vi "LSCI332 WaitSetpoint.vi"(0 "VISA Rsrc":refnum<visa-resource-name>="GPIB0::12::INSTR", 1 "ForceStop":refnum<vi>, 2 "Temp K":refnum<vi>, 3 "Heat":refnum<vi>, 5 "Wait Stab":bool=TRUE, 7 "SetPoint":dbl, 9 "Entré Activées":bool[](array[boolean])=[TRUE, FALSE], 11 "error in (no error)":errorcluster, 12 "Timeout":u32 caption="Timeout(s)", 13 "RangeK":dbl=0.01 min=0.01 max=100.0 step=0.01, 14 "InRangeTime":i32 caption="Req In Range Time(s)") -> (6 "TempOut (K)":dbl caption="Temp (K)", 8 "TempOut (S)":dbl, 15 "error out":errorcluster)   [LabVIEW 2019]
doc: "Ce VI écrit les paramètres limites de contrôle dans le contrôleur."
uses:
  <vilib>/Utility/error.llb/Error Cluster From Error Code.vi
  <userlib>/GenProg/ReadValByRefBool.vi
  <vilib>/ErrorRing/Error Ring.xnode
panel:
  in  "Open FP":bool
  in  "Force Stop":bool
  out "Elapsed Time(s)":u32 caption="Elapsed Time (s)" format="%<%H:%M>t"
  out "heating":bool
  out "Puissance(%)":dbl
  out "Échelle":u16
  out "Graphe XY":cluster{dbl[], dbl[]}[](graph)
  out "InRangeTimeOut":i32 caption="In Range Time (s)"
  out "In Range":bool
  in  "Boucle(1)":u32(ring) caption="Boucle" items=["Boucle 1", "Boucle 2"]
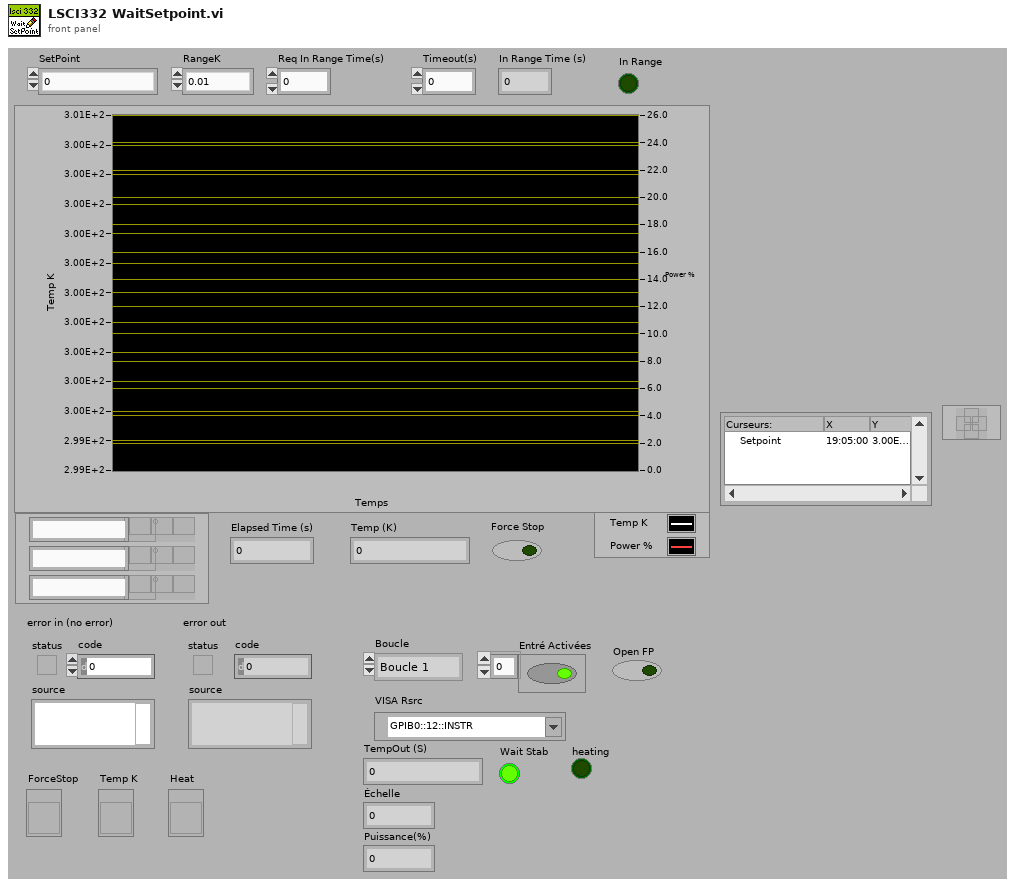
[diagram p1: front panel]
types:
  T1 = enum32{"Invalid", "Standard", "Closed", "Hidden", "Minimized", "Maximized"}
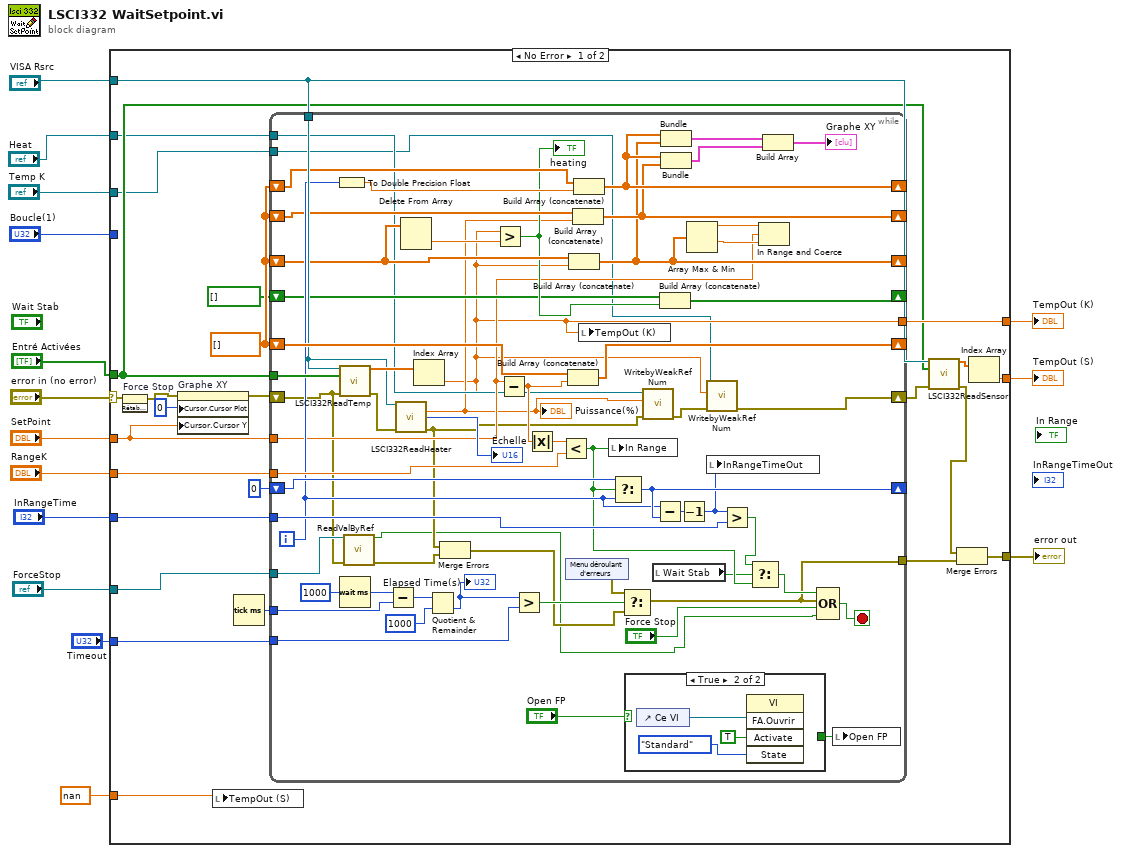
[diagram p0: block diagram]
diagram:
  n1 = case shown="No Error" "error in (no error)" {
    selector: "error in (no error)" -> [w22 w113]
    tunnel: "VISA Rsrc" -> [w34 _]
    tunnel: "Boucle(1)" -> [_ _]
    tunnel: [w30 w113] -> w13
    tunnel: "SetPoint" -> [w24 _]
    tunnel: "Entré Activées" -> [w31 _]
    tunnel: "Timeout" -> [w39 _]
    tunnel: "RangeK" -> [w38 _]
    tunnel: "InRangeTime" -> [w36 _]
    tunnel: [w35 _] -> w6
    tunnel: [w32 _] -> w5
    tunnel: nan ("TempOut (S)") -> [w28 _]
    tunnel: "ForceStop" -> [w16 _]
    tunnel: "Heat" -> [w18 _]
    tunnel: "Temp K" -> [w17 _]
    frame No Error {
      w27 = dbl[] []
      n2 = invoke on="Force Stop" class="Bool (strict)" method="RétablirValParDéfaut"(error in=w22) -> (error out=w21:errorcluster)  [unwired: 2 in, 2 out]
      n3 = property on="Graphe XY" class="GraphXY (strict)"(error in=w21, "Cursor.Cursor Plot"=0 ("Curseur.Tracé du curseur"), "Cursor.Cursor Y"=w24) -> (error out=w26:errorcluster)  [unwired: 1 in, 1 out]
      n4 = local write "TempOut (S)"(w28) -> ()
      n5 = Tick Count (ms)() -> (millisecond timer value=w40:u32)
      n6 = while {
        tunnel: w34 -> [w82]
        tunnel: w31 -> [w103]
        tunnel: w40 -> [w100]
        tunnel: w24 -> [w59]
        shift-right: [w101] -> _
        shift-left: w27 -> [w102]
        tunnel: w39 -> [w97]
        shift-right: [w45] -> w20
        shift-left: w26 -> [w56]
        shift-right: [w67] -> _
        shift-left: w27 -> [w70]
        tunnel: w38 -> [w90]
        shift-right: [w87] -> _
        shift-left: 0 -> [w80]
        tunnel: w36 -> [w85]
        tunnel: [w48] -> w35
        shift-right: [w75] -> _
        shift-left: w27 -> [w77]
        shift-right: [w74] -> _
        shift-left: w27 -> [w76]
        shift-right: [w66] -> _
        shift-left: bool[] [] -> [w65]
        tunnel: w16 -> [w57]
        tunnel: [w54] -> w19
        tunnel: w18 -> [w51]
        tunnel: w17 -> [w47]
        i -> [w79]
        stop <- w96 stop-if-true
        n7 = To Double Precision Float(number=w79) -> (double precision float=w78:dbl)
        n8 = call <userlib>:"LSCI332ReadTemp.vi"("VISA Rsrc"=w82, "Activées"=w103, "error in"=w56) -> ("Données"=w93:dbl[], "error out"=w83:errorcluster)  [unwired: 11 in]
        n9 = Wait (ms)(milliseconds to wait=u32 1000 ("attente (ms)")) -> (millisecond timer value=w88:u32)
        n10 = call-poly <userlib>:"ReadValByRef.vi"("Control Ref"=w57, "error in"=w56) -> ("Valeur"=w44:bool, "error out"=w53:errorcluster)  [unwired: 12 in]
        n11 = Subtract(x=w88, y=w100) -> (x-y=w99:u32)
        n12 = call <userlib>:"LSCI332ReadHeater.vi"("VISA Rsrc"=w82, "error in"=w83) -> ("Puissance(%)"=w50:dbl, "Échelle"=→"Échelle":u16, "error out"=w49:errorcluster)  [unwired: 10 in, 1 out]
        "Puissance(%)" <- w50
        n13 = Delete From Array(array=w70) -> (deleted portion=w69:dbl)  [unwired: 2 in, 1 out]
        n14 = Index Array(array=w93) -> (element=w48:dbl)  [unwired: 1 in]
        n15 = Quotient & Remainder(x=w99, y=u32 1000) -> (floor(x/y)=w64:u32)  [unwired: 1 out]
        "Elapsed Time(s)" <- w64
        n16 = Merge Errors(w49, w53) -> (w52:errorcluster)
        n17 = Greater?(x=w48, y=w69) -> (0:w68:bool)
        "heating" <- w68
        n18 = Subtract(x=w59, y=w48) -> (x-y=w92:dbl)
        n19 = Greater?(x=w64, y=w97) -> (0:w94:bool)
        n20 = Absolute Value(x=w92) -> (abs(x)=w91:dbl)
        n21 = Less?(x=w91, y=w90) -> (x < y?=w62:bool)
        n22 = xnode "Menu déroulant d'erreurs"() -> ("error out"=w95:errorcluster)
        n23 = Build Array (concatenate)(w102, w92) -> (w101:dbl[])
        n24 = Build Array (concatenate)(w70, w48) -> (w67:dbl[])
        n25 = Build Array (concatenate)(w76, w50) -> (w74:dbl[])
        n26 = Build Array (concatenate)(w77, w78) -> (w75:dbl[])
        n27 = local write "TempOut (K)"(w48) -> ()
        n28 = local write "In Range"(w62) -> ()
        n29 = Select(t=w80, s=w62, f=w79) -> (s? t:f=w87:i32)
        n30 = Select(t=w95, s=w94, f=w52) -> (s? t:f=w54:errorcluster)
        n31 = case shown="True" "Open FP" {
          selector: "Open FP" -> [w104 _]
          tunnel: [w104 _] -> w43
          frame False {
          }
          frame True {
            n32 = control-ref of="Ce VI"() -> (w107:refnum<vi>)
            n33 = invoke class="VI" method="FA.Ouvrir"(reference=w107, "Activate"=TRUE ("Activer ?"), "State"=T1."Standard" ("État")) -> ()  [unwired: 2 in, 5 out]
          }
        }
        n34 = call <userlib>:"WritebyWeakRefNum.vi"("error in"=w49, "Valeur"=w50, "Control Ref"=w51) -> ("error out"=w46:errorcluster)  [unwired: 8 in]
        n35 = local read "Wait Stab"() -> (w42:bool)
        n36 = Subtract(x=w79, y=w87) -> (x-y=w86:i32)
        n37 = Build Array (concatenate)(w65, w68) -> (w66:bool[])
        n38 = Bundle(w75, w67) -> (w72:cluster{dbl[], dbl[]})  [unwired: 1 in]
        n39 = Bundle(w75, w74) -> (w73:cluster{dbl[], dbl[]})  [unwired: 1 in]
        n40 = Decrement(x=w86) -> (x-1=w84:i32)
        n41 = Array Max & Min(array=w67) -> (max value=w61:dbl, min value=w60:dbl)  [unwired: 2 out]
        n42 = call <userlib>:"WritebyWeakRefNum.vi"("error in"=w46, "Valeur"=w48, "Control Ref"=w47) -> ("error out"=w45:errorcluster)  [unwired: 8 in]
        n43 = local write "InRangeTimeOut"(w84) -> ()
        n44 = Greater?(x=w84, y=w85) -> (0:w63:bool)
        n45 = Select(t=w63, s=w42, f=w62) -> (s? t:f=w58:bool)
        n46 = In Range and Coerce(upper limit=w61, x=w59, lower limit=w60) -> ()  [unwired: 2 out]
        n47 = Build Array(w72, w73) -> (→"Graphe XY":cluster{dbl[], dbl[]}[])
        n48 = Compound Arithmetic op=OR ("Opérateur arithmétique")(w58, w54, "Force Stop", w44) -> (w96:bool)
        n49 = local write "Open FP"(w43) -> ()
      }
      n50 = call <userlib>:"LSCI332ReadSensor.vi"("VISA Rsrc"=w34, "Activées"=w31, "error in"=w20) -> ("Données"=w33:dbl[], "error out"=w29:errorcluster)  [unwired: 11 in]
      n51 = Merge Errors(w29, w19) -> (w30:errorcluster)
      n52 = Index Array(array=w33) -> (element=w32:dbl)  [unwired: 1 in]
    }
    frame Error {
    }
  }
  "error out" <- w13
  "TempOut (K)" <- w6
  "TempOut (S)" <- w5
